vi "mxwScript_API_AddXMLOption.vi"(8 "error in (no error)":errorcluster, 9 "tag text":string, 10 "tag":string, 11 "input":string) -> (0 "error out":errorcluster, 3 "encoded output":string)   [LabVIEW 2017]
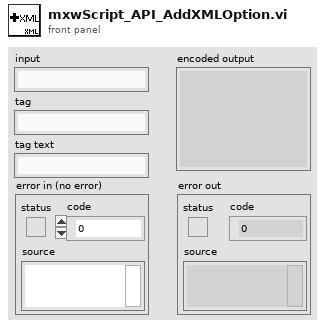
[diagram p1: front panel]
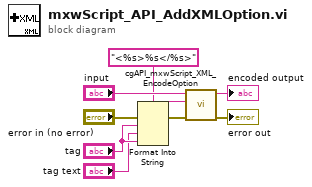
[diagram p0: block diagram]
diagram:
  n1 = Format Into String(format string="<%s>%s</%s>", error in="error in (no error)", "tag", "tag text", "tag") -> (resulting string=w4:string, error out=w5:errorcluster)  [unwired: 1 in]
  n2 = call "cgAPI_mxwScript_XML_EncodeOption.vi"("error in (no error)"=w5, "otherXML"=w4, "normalTextString"="input") -> ("error out"=→"error out":errorcluster, "encodedString"=→"encoded output":string)  [unwired: 7 out]
